vi "8-Line.vi"(0 "Line 8":string, 1 "Line 7":string, 2 "Line 6":string, 4 "Line 5":string, 6 "Line 4":string, 8 "Line 3":string, 9 "Line 2":string, 10 "Line 1":string, 11 "NXT":T1={"error"={"status"=FALSE, "code"=0, "source"=""}, "address"="", "NXT #"=0, "Show Error"=FALSE, "Connection"=4} {"Connection" items=["USB", "Bluetooth", "USB then Bluetooth", "Last Connection", "Preference"]}) -> (3 "NXT 2":T1={"error"={"status"=FALSE, "code"=0, "source"=""}, "address"="", "NXT #"=0, "Show Error"=FALSE, "Connection"=4} {"Connection" items=["USB", "Bluetooth", "USB then Bluetooth", "Last Connection", "Preference"]})   [LabVIEW 2009]
uses:
  <vilib>/NXT/Subs/LVHSConnector.ctl
  <vilib>/NXT/Dual Mode Library/Display/drawText.vi
panel:
  # "mindsensors.com\nCopyright (c) 2009 by mindsensors.com\nEmail: info (<at>) mindsensors (<dot>) com\n\nThis program is free software. You can redistribute it and/or modify\nit under the terms of the GNU General Public License as published by\nthe Free Software Foundation; version 3 of the License.\nRead the license at: http://www.gnu.org/licenses/gpl.txt"
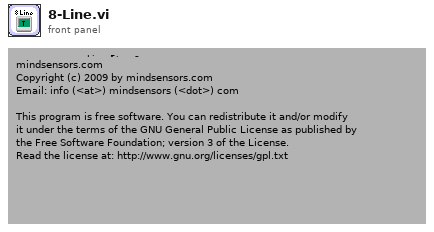
[diagram p1: front panel]
types:
  T1 = typedef "LVHSConnector.ctl" = cluster{"error":errorcluster, "address":string, "NXT #":i32, "Show Error":bool, "Connection":u16}
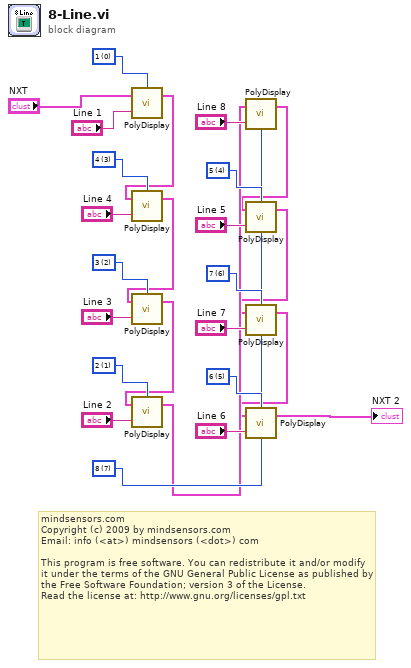
[diagram p0: block diagram]
diagram:
  w11 = i16 7 items=["1", "2", "3", "4", "5", "6", "7", "8"] ("Line")
  w13 = i16 6 items=["1", "2", "3", "4", "5", "6", "7", "8"] ("Line")
  w15 = i16 5 items=["1", "2", "3", "4", "5", "6", "7", "8"] ("Line")
  w17 = i16 4 items=["1", "2", "3", "4", "5", "6", "7", "8"] ("Line")
  w19 = i16 3 items=["1", "2", "3", "4", "5", "6", "7", "8"] ("Line")
  w21 = i16 2 items=["1", "2", "3", "4", "5", "6", "7", "8"] ("Line")
  w23 = i16 1 items=["1", "2", "3", "4", "5", "6", "7", "8"] ("Line")
  w25 = i16 0 items=["1", "2", "3", "4", "5", "6", "7", "8"] ("Line")
  # "mindsensors.com\nCopyright (c) 2009 by mindsensors.com\nEmail: info (<at>) mindsensors (<dot>) com\n\nThis program is free software. You can redistribute it and/or modify\nit under the terms of the GNU General Public License as published by\nthe Free Software Foundation; version 3 of the License.\nRead the license at: http://www.gnu.org/licenses/gpl.txt"
  n1 = call-poly <vilib>:"PolyDisplay.vi"("Text"="Line 1", "NXT"="NXT", "Line"=w25) -> ("NXT"=w8:T1)  [unwired: 1 in]
  n2 = call-poly <vilib>:"PolyDisplay.vi"("Text"="Line 4", "NXT"=w8, "Line"=w19) -> ("NXT"=w7:T1)  [unwired: 1 in]
  n3 = call-poly <vilib>:"PolyDisplay.vi"("Text"="Line 3", "NXT"=w7, "Line"=w21) -> ("NXT"=w6:T1)  [unwired: 1 in]
  n4 = call-poly <vilib>:"PolyDisplay.vi"("Text"="Line 2", "NXT"=w6, "Line"=w23) -> ("NXT"=w5:T1)  [unwired: 1 in]
  n5 = call-poly <vilib>:"PolyDisplay.vi"("Text"="Line 8", "NXT"=w5, "Line"=w11) -> ("NXT"=w4:T1)  [unwired: 1 in]
  n6 = call-poly <vilib>:"PolyDisplay.vi"("Text"="Line 5", "NXT"=w4, "Line"=w17) -> ("NXT"=w3:T1)  [unwired: 1 in]
  n7 = call-poly <vilib>:"PolyDisplay.vi"("Text"="Line 7", "NXT"=w3, "Line"=w13) -> ("NXT"=w2:T1)  [unwired: 1 in]
  n8 = call-poly <vilib>:"PolyDisplay.vi"("Text"="Line 6", "NXT"=w2, "Line"=w15) -> ("NXT"=→"NXT 2":T1)  [unwired: 1 in]
